vi "Get Queue Reference.vi"(8 "error in (no error)":errorcluster) -> (0 "error out":errorcluster, 2 "created new?":bool, 3 "Message Queue":refnum<queue>)   [LabVIEW 2016, in "AssertEngine.lvlib"]
uses:
  AssertEngine.lvlib
  Classes/External Msg.lvclass
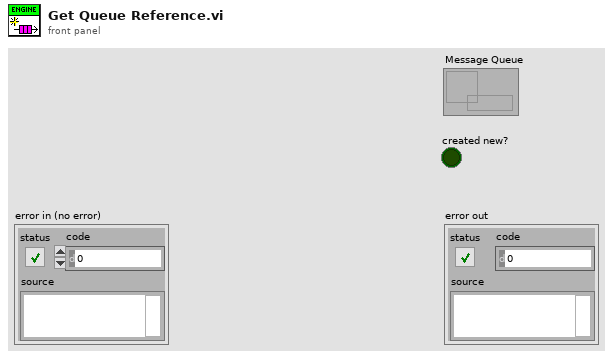
[diagram p1: front panel]
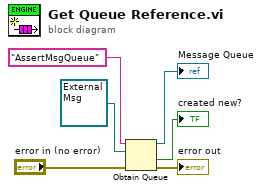
[diagram p0: block diagram]
diagram:
  n1 = Obtain Queue(name (unnamed)="AssertMsgQueue", element data type=refnum<class "External Msg.lvclass"> refnum ("AssertEngine.lvlib:External Msg.lvclass"), error in (no error)="error in (no error)") -> (queue out=→"Message Queue":refnum<queue>, created new?=→"created new?":bool, error out=→"error out":errorcluster)  [unwired: 2 in]
